vi "Scan ALL.vi"() -> ()   [LabVIEW 2016, in "SetUp VIs.lvlib"]
uses:
  SetUp VIs.lvlib
  Controls/Enum for Instrument Finder State Machine.ctl
  Device/Generic Device.lvclass
  C:/Users/Jlarrieux/Documents/LabView Git Repo/Generic Instrument/Subpanel Insertion/Subpanel Inserter.lvclass
  C:/Program Files (x86)/National Instruments/LabVIEW 2016/vi.lib/ActorFramework/Actor/Actor.lvclass
  Controls/Instrument ID Object.ctl
  Generic Instrument/Generic Instrument.lvclass
panel:
  out "Array of Instruments":refnum<class "Generic Instrument.lvclass">[](array[class])
  in  "List of Instruments":T1[](array[typedef])
  out "Cancel Out":bool
  out "error IO":errorcluster
  out "big i":i32
  in  "Rescan":bool
  in  "Done":bool
  in  "Cancel":bool
  out "find list":string[](array[string])
  out "specific error cleared?":bool
  out "Array":errorcluster[](array[cluster])
  out "Array 2":string[](array[string])
  in  "error in (no error)":errorcluster
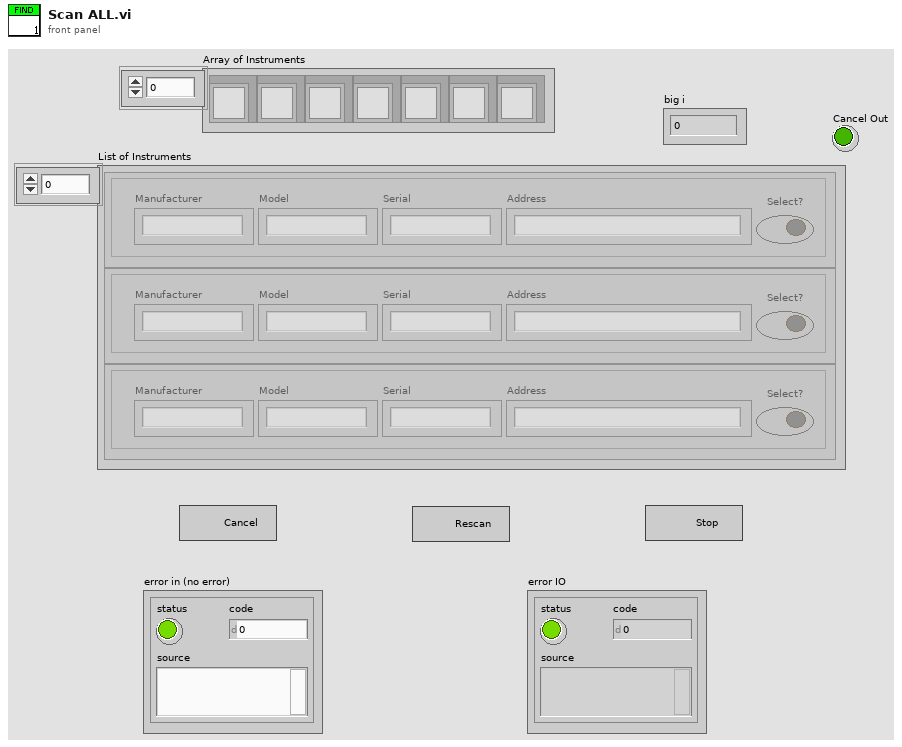
[diagram p1: front panel]
types:
  T1 = typedef "Instrument ID Object.ctl" = cluster{"Manufacturer":string, "Model":string, "Serial":string, "Address":string, "Select?":bool}
  T2 = typedef "Enum for Instrument Finder State Machine.ctl" = enum16{"Wait", "Scan", "Done"}
  T3 = cluster{"Manufacturer":string, "Model":string, "Serial":string, "Address":string, "Boolean":bool}[]
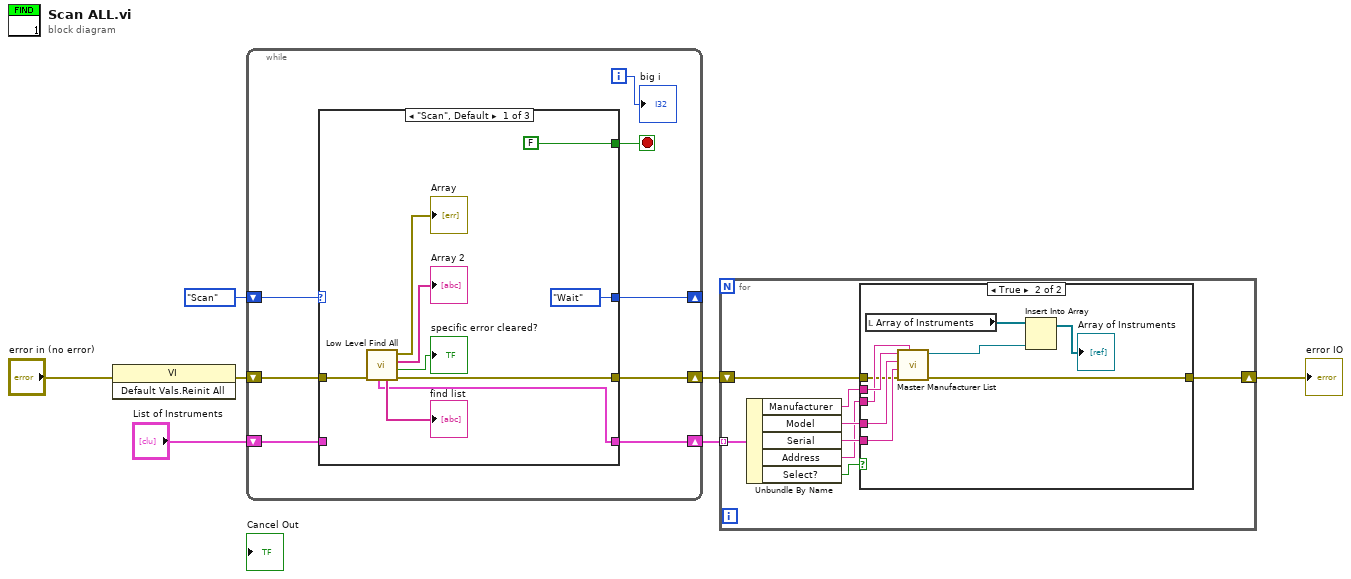
[diagram p0: block diagram]
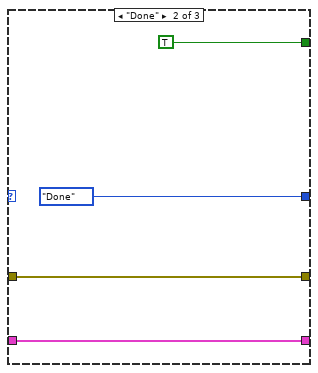
[diagram p3: hidden frame]
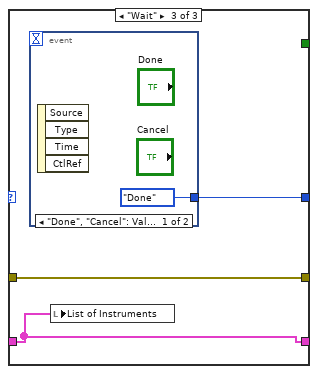
[diagram p4: hidden frame]
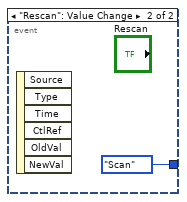
[diagram p5: hidden frame]
diagram:
  n1 = invoke class="VI" method="Default Vals.Reinit All"(error in="error in (no error)") -> (error out=w6:errorcluster)  [unwired: 2 in, 2 out]
  n2 = while {
    shift-right: [w13] -> w2
    shift-left: w6 -> [w15]
    shift-right: [w10] -> _
    shift-left: Enum_for_Instrument_Finder_State_Machine."Scan" ("Enum") -> [w12]
    shift-right: [w9] -> w3
    shift-left: "List of Instruments" -> [w8]
    i -> [w14]
    stop <- w11 stop-if-true
    n3 = case shown="\"Scan\", Default" w12 {
      tunnel: w15 -> [w24 w26 w30]
      tunnel: [w23 w26 w30] -> w13
      tunnel: [FALSE TRUE _] -> w11
      tunnel: [Enum_for_Instrument_Finder_State_Machine."Wait" ("Enum") Enum_for_Instrument_Finder_State_Machine."Done" ("Enum") w31] -> w10
      tunnel: [w17 w25 w29] -> w9
      tunnel: w8 -> [_ w25 w29]
      frame "Scan", Default {
        n4 = call "Low Level Find All.vi"("error in (no error)"=w24) -> ("error out"=w23:errorcluster, "specific error cleared?"=→"specific error cleared?":bool, "Array 2"=→"Array 2":string[], "Array"=→"Array":errorcluster[], "find list"=→"find list":string[], "List of Instruments"=w17:T3)  [unwired: 4 in, 1 out]
      }
      frame "Done" {
      }
      frame "Wait" {
        n5 = event shown="[0] \"Done\", \"Cancel\": Value Change" {
          selector: _ -> [_ _]
          dyn-events: _ -> [_ _]
          timeout: _ -> [_ _]
          tunnel: [Enum_for_Instrument_Finder_State_Machine."Done" ("Enum") Enum_for_Instrument_Finder_State_Machine."Scan" ("Enum")] -> w31
          event "Done", "Cancel": Value Change {
            n6 = event-data() -> ()  [unwired: 1 in, 4 out]
          }
          event "Rescan": Value Change {
            n7 = event-data() -> ()  [unwired: 1 in, 6 out]
          }
        }
        n8 = local write "List of Instruments"(w29) -> ()
      }
    }
    "big i" <- w14
  }
  n9 = for {
    tunnel: w3 -> [w41] mode=indexing
    shift-right: [w34] -> w1
    shift-left: w2 -> [w35]
    n10 = Unbundle By Name(w41) -> ("Manufacturer"=w39:string, "Model"=w38:string, "Serial"=w37:string, "Address"=w36:string, "Select?"=w40:bool)
    n11 = case shown="True" w40 {
      tunnel: w39 -> [_ w51]
      tunnel: w38 -> [_ w50]
      tunnel: w37 -> [_ w49]
      tunnel: w36 -> [_ w48]
      tunnel: w35 -> [w42 w47]
      tunnel: [w42 w46] -> w34
      frame False {
      }
      frame True {
        n12 = local read "Array of Instruments"() -> (w45:refnum<class "Generic Instrument.lvclass">[])
        n13 = call "Master Manufacturer List.vi"("VISA resource name"=w48, "error in"=w47, "Serial"=w49, "Model In"=w50, "Manufacturer"=w51) -> ("error out"=w46:errorcluster, "Generic Device.lvlib:Generic Device.lvclass"=w44:refnum<class "Generic Device.lvclass">)  [unwired: 5 in]
        n14 = Insert Into Array(array=w45, new element=w44) -> (→"Array of Instruments":refnum<class "Generic Instrument.lvclass">[])  [unwired: 1 in]
      }
    }
  }
  "error IO" <- w1
